vi "FromFrequncy.vi"(0 "A":dbl, 1 "Z":dbl, 2 "F":dbl, 3 "Rm":dbl, 4 "UECR":dbl, 5 "HARM":dbl=3.0, 6 "Rextr":dbl=1.78) -> (7 "Uinfl":dbl, 9 "Ubender":dbl, 11 "UIAT":dbl, 12 "Udef":dbl, 13 "Uinj":dbl, 14 "A/Z":dbl, 15 "E (MeV)":dbl, 16 "MeV/u":dbl, 17 "B0(kGs)":dbl, 18 "B0(T)":dbl, 19 "Im":dbl)   [LabVIEW 2018, in "Class 2.lvclass"]
uses:
  Class 2.lvclass
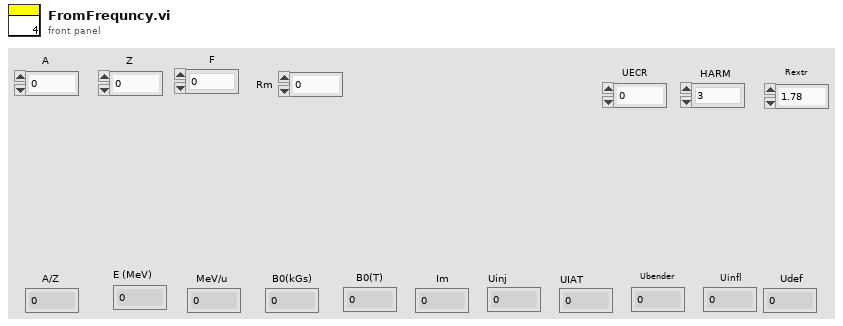
[diagram p1: front panel]
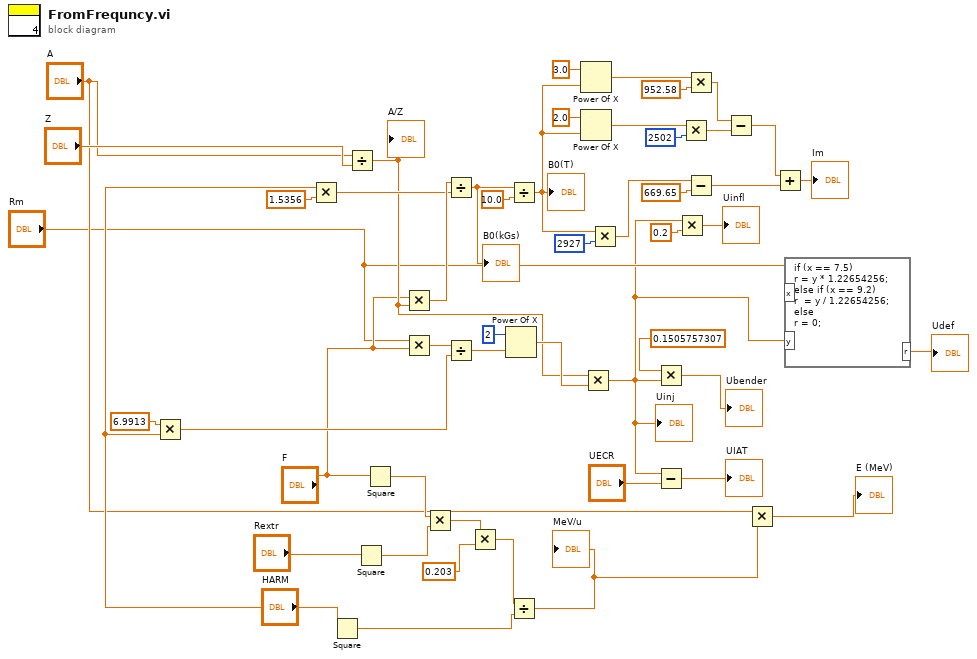
[diagram p0: block diagram]
diagram:
  n1 = Multiply(x=6.9913, y="HARM") -> (x*y=w29:dbl)
  n2 = Multiply(x="HARM", y=1.5356) -> (x*y=w46:dbl)
  n3 = Square(x="HARM") -> (x^2=w8:dbl)
  n4 = Divide(x="A", y="Z") -> (x/y=w19:dbl)
  "A/Z" <- w19
  n5 = Square(x="Rextr") -> (x^2=w13:dbl)
  n6 = Square(x="F") -> (x^2=w14:dbl)
  n7 = Multiply(x="F", y=w19) -> (x*y=w47:dbl)
  n8 = Multiply(x="Rm", y="F") -> (x*y=w30:dbl)
  n9 = Multiply(x=w14, y=w13) -> (x*y=w12:dbl)
  n10 = Divide(x=w47, y=w46) -> (x/y=w17:dbl)
  "B0(kGs)" <- w17
  n11 = Divide(x=w30, y=w29) -> (x/y=w28:dbl)
  n12 = Multiply(x=w12, y=0.203) -> (x*y=w9:dbl)
  n13 = Power Of X(1:w28, 2:2) -> (0:w26:dbl)
  n14 = Divide(x=w17, y=10.0) -> (x/y=w18:dbl)
  "B0(T)" <- w18
  n15 = Divide(x=w9, y=w8) -> (x/y=w7:dbl)
  "MeV/u" <- w7
  n16 = Power Of X(1:w18, 2:3.0 ("y")) -> (0:w43:dbl)
  n17 = Power Of X(1:w18, 2:2.0 ("y")) -> (0:w41:dbl)
  n18 = Multiply(x=w19, y=w26) -> (x*y=w2:dbl)
  "Uinj" <- w2
  n19 = Multiply(x=w18, y=2927) -> (x*y=w35:dbl)
  n20 = Multiply(x=0.1505757307, y=w2) -> (x*y=→"Ubender":dbl)
  n21 = Subtract(x=w2, y="UECR") -> (x-y=→"UIAT":dbl)
  n22 = Multiply(x=w2, y=0.2) -> (x*y=→"Uinfl":dbl)
  n23 = Multiply(x=w41, y=2502) -> (x*y=w36:dbl)
  n24 = Multiply(x=w43, y=952.58) -> (x*y=w37:dbl)
  n25 = Subtract(x=w35, y=669.65) -> (x-y=w32:dbl)
  n26 = Subtract(x=w37, y=w36) -> (x-y=w33:dbl)
  n27 = Multiply(x="A", y=w7) -> (x*y=→"E (MeV)":dbl)
  n28 = Add(x=w33, y=w32) -> (x+y=→"Im":dbl)
  n29 = formula code="if (x == 7.5)\nr = y * 1.22654256;\nelse if (x == 9.2)\nr  = y / 1.22654256;\nelse\nr = 0;"("x"="Rm", "y"=w2) -> ("r"=→"Udef":dbl)
